vi "Write Range.vi"(8 "error in (no error)":errorcluster, 10 "Range":T1, 11 "Scanner in":refnum<class "Scanner.lvclass">) -> (0 "error out":errorcluster, 2 "# Points":u32, 3 "Scanner out":refnum<class "Scanner.lvclass">)   [LabVIEW 2009, in "Scanner.lvclass"]
doc: "Set the Range of this Scanner to the Range of another Scanner."
uses:
  Scanner.lvclass
  Range.ctl
  Scanner.lvclass/Scanner.ctl
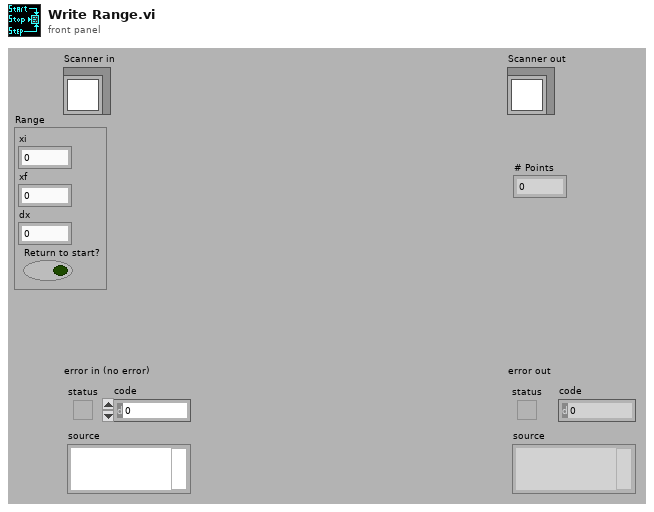
[diagram p1: front panel]
types:
  T1 = typedef "Scanner.lvclass/Range.ctl" = cluster{"xi":dbl, "xf":dbl, "dx":dbl, "Return to start?":bool}
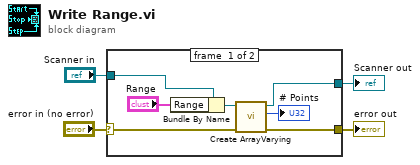
[diagram p0: block diagram]
diagram:
  n1 = case shown="No Error" "error in (no error)" {
    selector: "error in (no error)" -> [w10 w13]
    tunnel: [w9 w13] -> w3
    tunnel: [w7 w12] -> w1
    tunnel: "Scanner in" -> [w11 w12]
    frame #0 {
      n2 = Bundle By Name(cluster=w11, "Range"="Range") -> (w8:refnum<class "Scanner.lvclass">)
      n3 = call "Create ArrayVarying.vi"("error in (no error)"=w10, "Scanner.lvclass"=w8) -> ("error out"=w9:errorcluster, "# Points"=→"# Points":u32, "Scanner.lvclass out"=w7:refnum<class "Scanner.lvclass">)  [unwired: 7 out]
    }
    frame #1 {
    }
  }
  "error out" <- w3
  "Scanner out" <- w1
